vi "GoHome.vi"(2 "error in":errorcluster, 3 "Axis":enum16{"Z", "Y", "X"}(ring), 4 "Speed (counts/s)":i32=40000, 5 "connection refnum in":refnum<k5>) -> (0 "error out":errorcluster, 1 "connection refnum out":refnum<k5>)   [LabVIEW 2023]
doc: "Use the homing command \"macro\" to move the device to its home position\nSpeed counts is defaulted to 40,000 which is about 2mm/s"
uses:
  GlobalVarsNetwork.vi
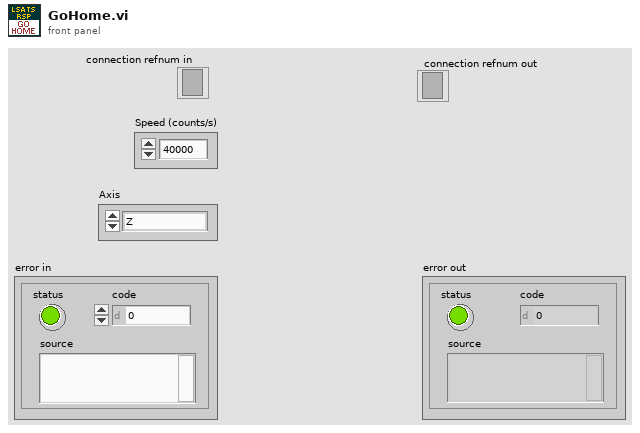
[diagram p1: front panel]
types:
  T1 = cluster{"XY_IP_ADDRESS":string, "Z_IP_ADDRESS":string, "Port":u16, "connection refnum x,y":refnum<k5>, "connection refnum z":refnum<k5>}
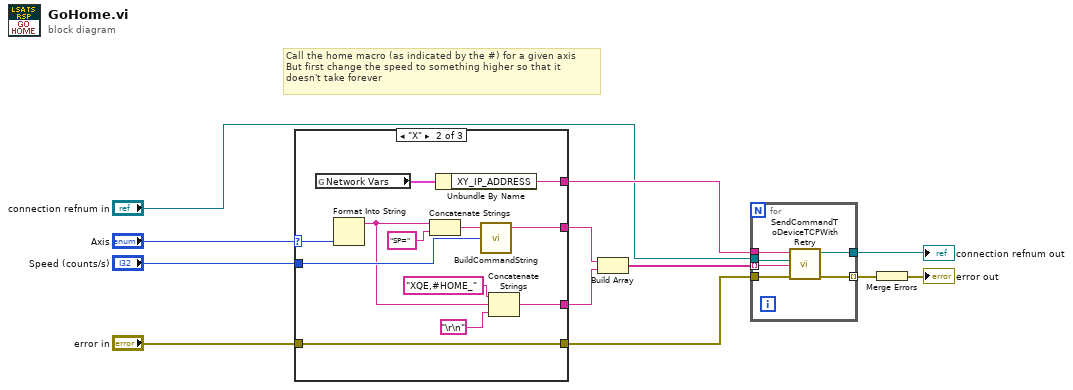
[diagram p0: block diagram]
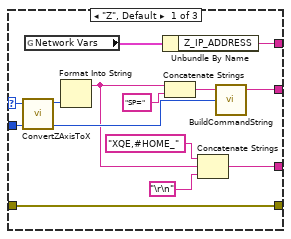
[diagram p2: hidden frame]
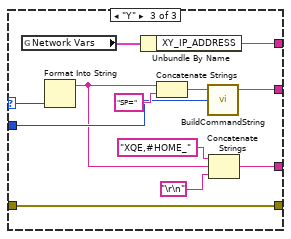
[diagram p3: hidden frame]
diagram:
  # "Call the home macro (as indicated by the #) for a given axis\nBut first change the speed to something higher so that it \ndoesn't take forever"
  n1 = case shown="\"X\"" "Axis" {
    selector: "Axis" -> [w15 w27 w39]
    tunnel: [w24 w33 w48] -> w10
    tunnel: [w22 w32 w44] -> w7
    tunnel: "error in" -> [w20 w37 w47]
    tunnel: [w20 w37 w47] -> w12
    tunnel: "Speed (counts/s)" -> [w17 w29 w41]
    tunnel: [w16 w28 w40] -> w8
    frame "Z", Default {
      n2 = call "ConvertZAxisToX.vi"("Axis in"=w15) -> ("Axis out"=w14:enum16{"Z", "Y", "X"})  [unwired: 6 in]
      n3 = global read "GlobalVarsNetwork.vi" "Network Vars"() -> (w25:T1)
      n4 = Format Into String(w14) -> (resulting string=w13:string)  [unwired: 3 in, 1 out]
      n5 = Unbundle By Name(w25) -> ("Z_IP_ADDRESS"=w24:string)
      n6 = Concatenate Strings(w13, "SP=") -> (w19:string)
      n7 = Concatenate Strings("XQE,#HOME_", w13, "\r\n") -> (w22:string)
      n8 = call "BuildCommandString.vi"("Numeric Value"=w17, "Command"=w19) -> ("Result"=w16:string)  [unwired: 2 in, 1 out]
    }
    frame "X" {
      n9 = global read "GlobalVarsNetwork.vi" "Network Vars"() -> (w36:T1)
      n10 = Format Into String(w27) -> (resulting string=w26:string)  [unwired: 3 in, 1 out]
      n11 = Concatenate Strings(w26, "SP=") -> (w30:string)
      n12 = Unbundle By Name(w36) -> ("XY_IP_ADDRESS"=w33:string)
      n13 = call "BuildCommandString.vi"("Numeric Value"=w29, "Command"=w30) -> ("Result"=w28:string)  [unwired: 2 in, 1 out]
      n14 = Concatenate Strings("XQE,#HOME_", w26, "\r\n") -> (w32:string)
    }
    frame "Y" {
      n15 = global read "GlobalVarsNetwork.vi" "Network Vars"() -> (w49:T1)
      n16 = Format Into String(w39) -> (resulting string=w38:string)  [unwired: 3 in, 1 out]
      n17 = Unbundle By Name(w49) -> ("XY_IP_ADDRESS"=w48:string)
      n18 = Concatenate Strings(w38, "SP=") -> (w42:string)
      n19 = call "BuildCommandString.vi"("Numeric Value"=w41, "Command"=w42) -> ("Result"=w40:string)  [unwired: 2 in, 1 out]
      n20 = Concatenate Strings("XQE,#HOME_", w38, "\r\n") -> (w44:string)
    }
  }
  n21 = Build Array(w8, w7) -> (w6:string[])
  n22 = for {
    tunnel: w10 -> [w53]
    tunnel: w6 -> [w52] mode=indexing
    tunnel: w12 -> [w54]
    tunnel: [w55] -> w5 mode=indexing
    tunnel: [w51] -> w3
    tunnel: "connection refnum in" -> [w50]
    n23 = call "SendCommandToDeviceTCPWithRetry.vi"("error in"=w54, "str command"=w52, "connection refnum in"=w50, "IP address"=w53) -> ("error out"=w55:errorcluster, "connection refnum out"=w51:refnum<k5>)  [unwired: 4 in, 2 out]
  }
  "connection refnum out" <- w3
  n24 = Merge Errors(w5) -> (→"error out":errorcluster)
